vi "Parameters_file_v01.vi"(4 "Additional text":string, 5 "actual sample rate array":dbl[](array[numeric]), 6 "actualSamples array":i32[](array[numeric]), 7 "Files name array":string[](array[string]), 8 "File location":path, 9 "Record":bool) -> (0 "Full text":string)   [LabVIEW 2013]
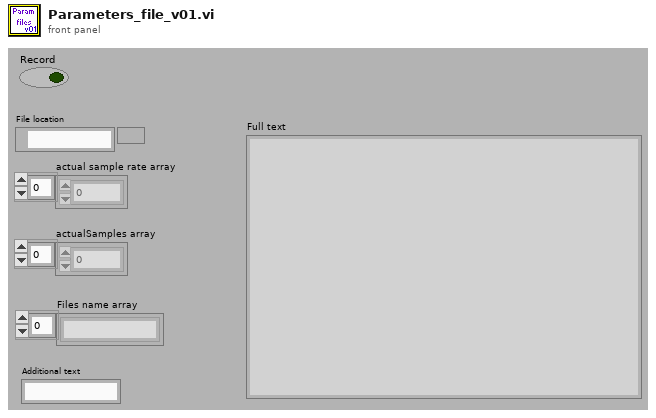
[diagram p1: front panel]
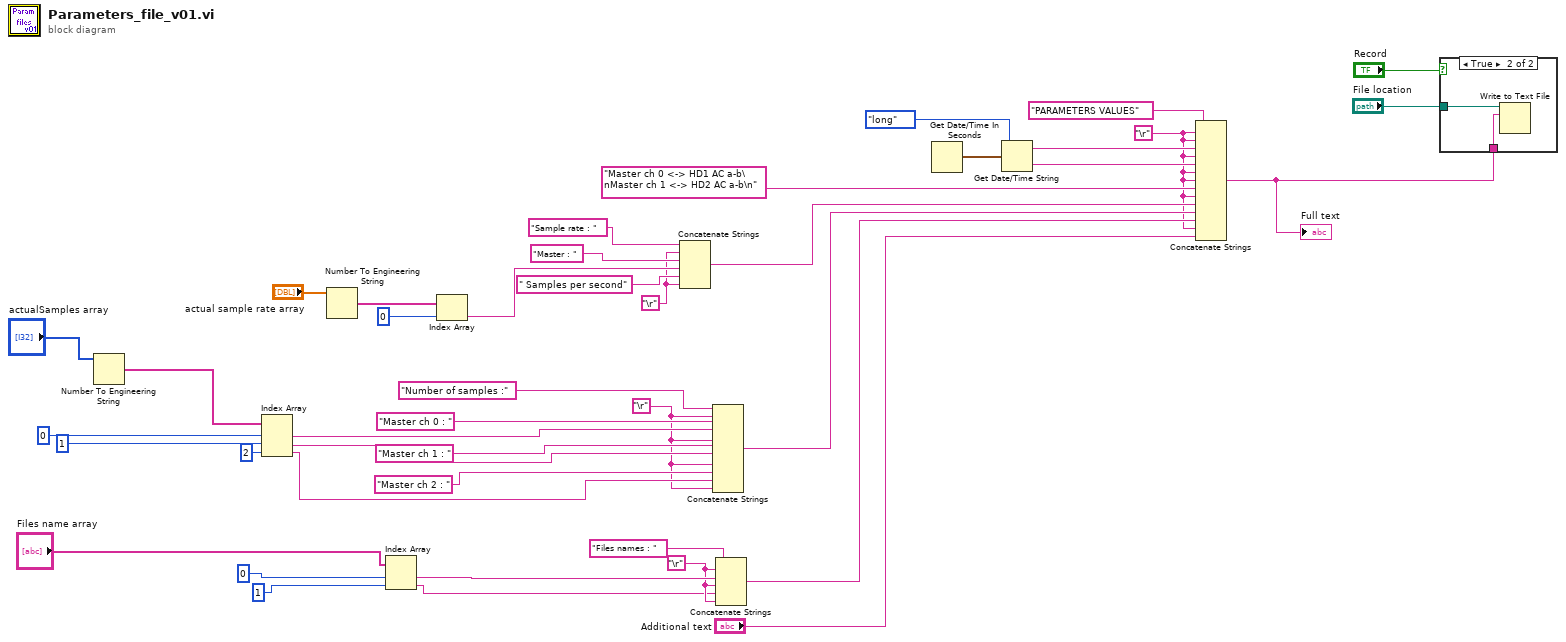
[diagram p0: block diagram]
diagram:
  w14 = "\r"
  w1 = "\r"
  w8 = "\r"
  w5 = "\r"
  n1 = Number To Engineering String(4:"actualSamples array") -> (0:w32:string[])  [unwired: 3 out]
  n2 = Index Array(array=w32, index #1=0 ("index"), index #2=1 ("index"), index #3=2 ("index")) -> (element #1=w26:string, element #2=w24:string, element #3=w2:string)
  n3 = Number To Engineering String(4:"actual sample rate array") -> (0:w19:string[])  [unwired: 3 out]
  n4 = Index Array(array="Files name array", index #1=0 ("index"), index #2=1 ("index")) -> (element #1=w9:string, element #2=w7:string)
  n5 = Index Array(array=w19, index=0) -> (element=w16:string)
  n6 = Concatenate Strings("Sample rate : " ("string"), w14, "Master : " ("string"), w16, " Samples per second" ("string"), w14) -> (w23:string)
  n7 = Concatenate Strings("Number of samples :" ("string"), w1, "Master ch 0 : " ("string"), w26, w1, "Master ch 1 : " ("string"), w24, w1, "Master ch 2 : " ("string"), w2, w1) -> (w22:string)
  n8 = Concatenate Strings("Files names : " ("string"), w8, w9, w8, w7, w8) -> (w21:string)
  n9 = Get Date/Time In Seconds() -> (seconds since 1Jan1904=w39:timestamp)
  n10 = Get Date/Time String(date format (0)=enum16{"short", "long", "abbreviated"}."long", seconds (now)=w39) -> (date string=w36:string, time string=w38:string)  [unwired: 1 out]
  n11 = Concatenate Strings("PARAMETERS VALUES" ("string"), w5, w5, w36, w5, w38, w5, w5, "Master ch 0 <-> HD1 AC a-b\nMaster ch 1 <-> HD2 AC a-b\n", w5, w23, w22, w21, w5, "Additional text") -> (w40:string)
  "Full text" <- w40
  n12 = case shown="True" "Record" {
    tunnel: "File location" -> [_ w44]
    tunnel: w40 -> [_ w43]
    frame False {
    }
    frame True {
      n13 = Write to Text File(file (use dialog)=w44, text=w43) -> ()  [unwired: 1 in, 4 out]
    }
  }
